vi "main.vi"(11 "Camera":refnum<queue>) -> ()   [LabVIEW 2024, in "RSeries_CAM.lvlib"]
uses:
  RSeries_CAM.lvlib
  ARCH/Message Queue/Message Cluster.ctl
  SRC/SUBVIS/RSeries_CAM.lvclass
  SRC/SUBVIS/RSeries_CAM.lvclass/RSeries_CAM.ctl
  SRC/CTRLS/CAM module Data.ctl
  CTRLS/GLB_VAR.vi
  ARCH/Message Queue/Message Queue.lvlib
panel:
  out "error out 5":errorcluster
  out "error out 4":errorcluster
  out "error out 3":errorcluster
  out "error out":errorcluster
  out "local stop":bool
  out "data out":string
  out "error out 2":errorcluster
  in  "Port 3":u32=3000
  out "RSeries_CAM out":refnum<class "RSeries_CAM.lvclass">
  out "Array":string[](array[string])
  in  "Send Vars":bool
  in  "Cluster":T1
  out "Response":string
  out "Connection status":bool
  in  "Port 2":u32=3001
  in  "Send Command":bool
  in  "Connect":bool
  in  "Command":string
  in  "IP":string="192.168.250.5"
  in  "RSeries_CAM.lvlib:RSeries_CAM.lvclass":refnum<class "RSeries_CAM.lvclass">
  in  "stop":bool
  in  "UNIT TESTING":bool
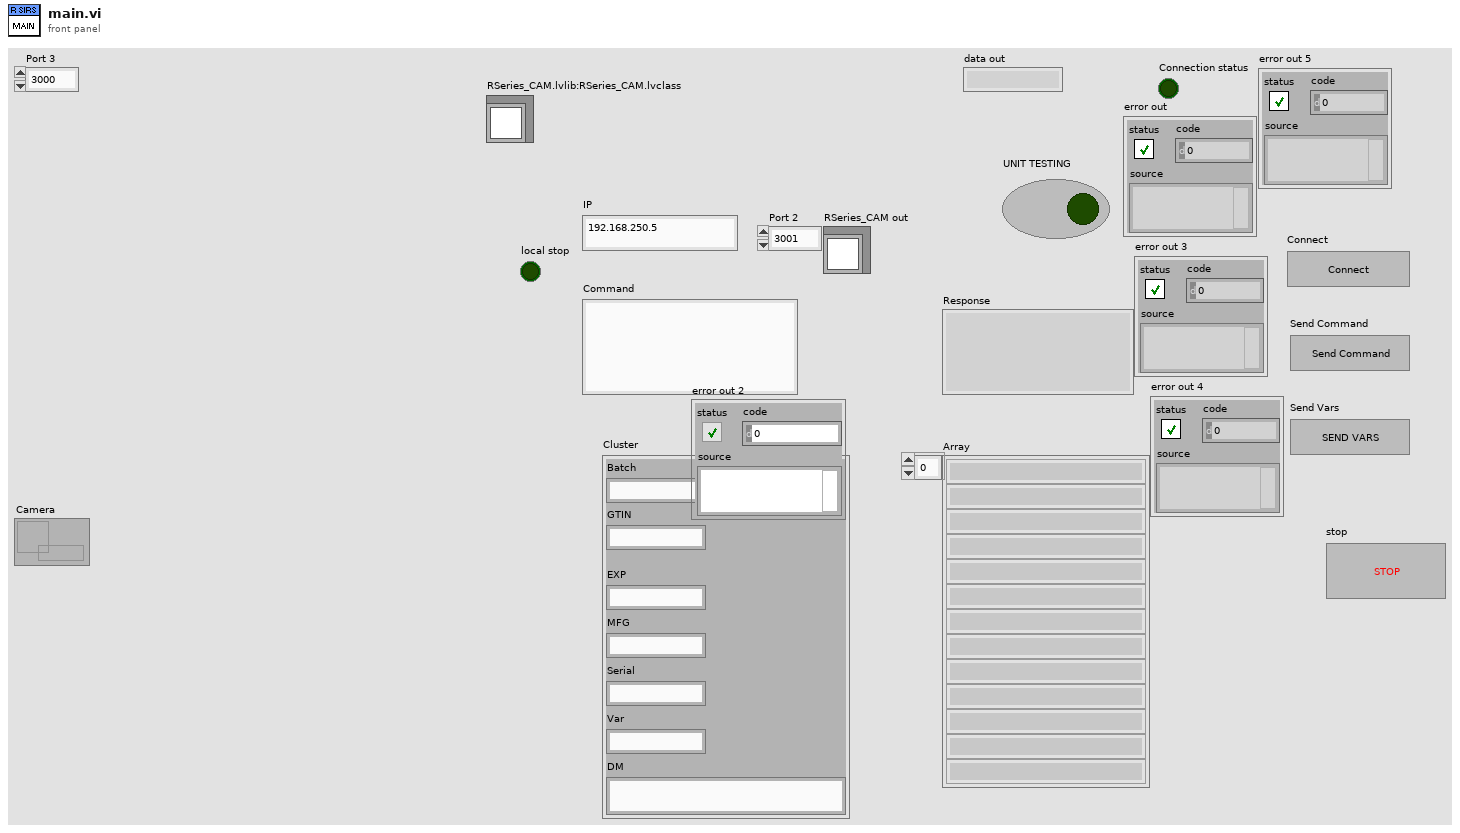
[diagram p1: front panel]
types:
  T1 = cluster{"Batch":string, "GTIN":string, "EXP":string, "MFG":string, "Serial":string, "Var":string, "DM":string}
  T2 = typedef "CAM module Data.ctl" = cluster{"IP":string, "sending Port ":u32, "BatchData":refnum<vi>, "Recieveing Port":u32, "Caller Quue":refnum<queue>}
  T3 = cluster{"Subscriber message":string, "Subscriber queue":refnum<queue>}
  T4 = typedef "Message Queue.lvlib/Message Cluster.ctl" = cluster{"Message":string, "Message Data":variant}
  T5 = enum16{"Standard", "Buffered", "CRLF", "Immediate"}
  T6 = enum16{"Init SRL Buffer", "Insert SRL in Buffer", "Insert SRL Status", "Remove SRL from Buffer", "pop serial"}
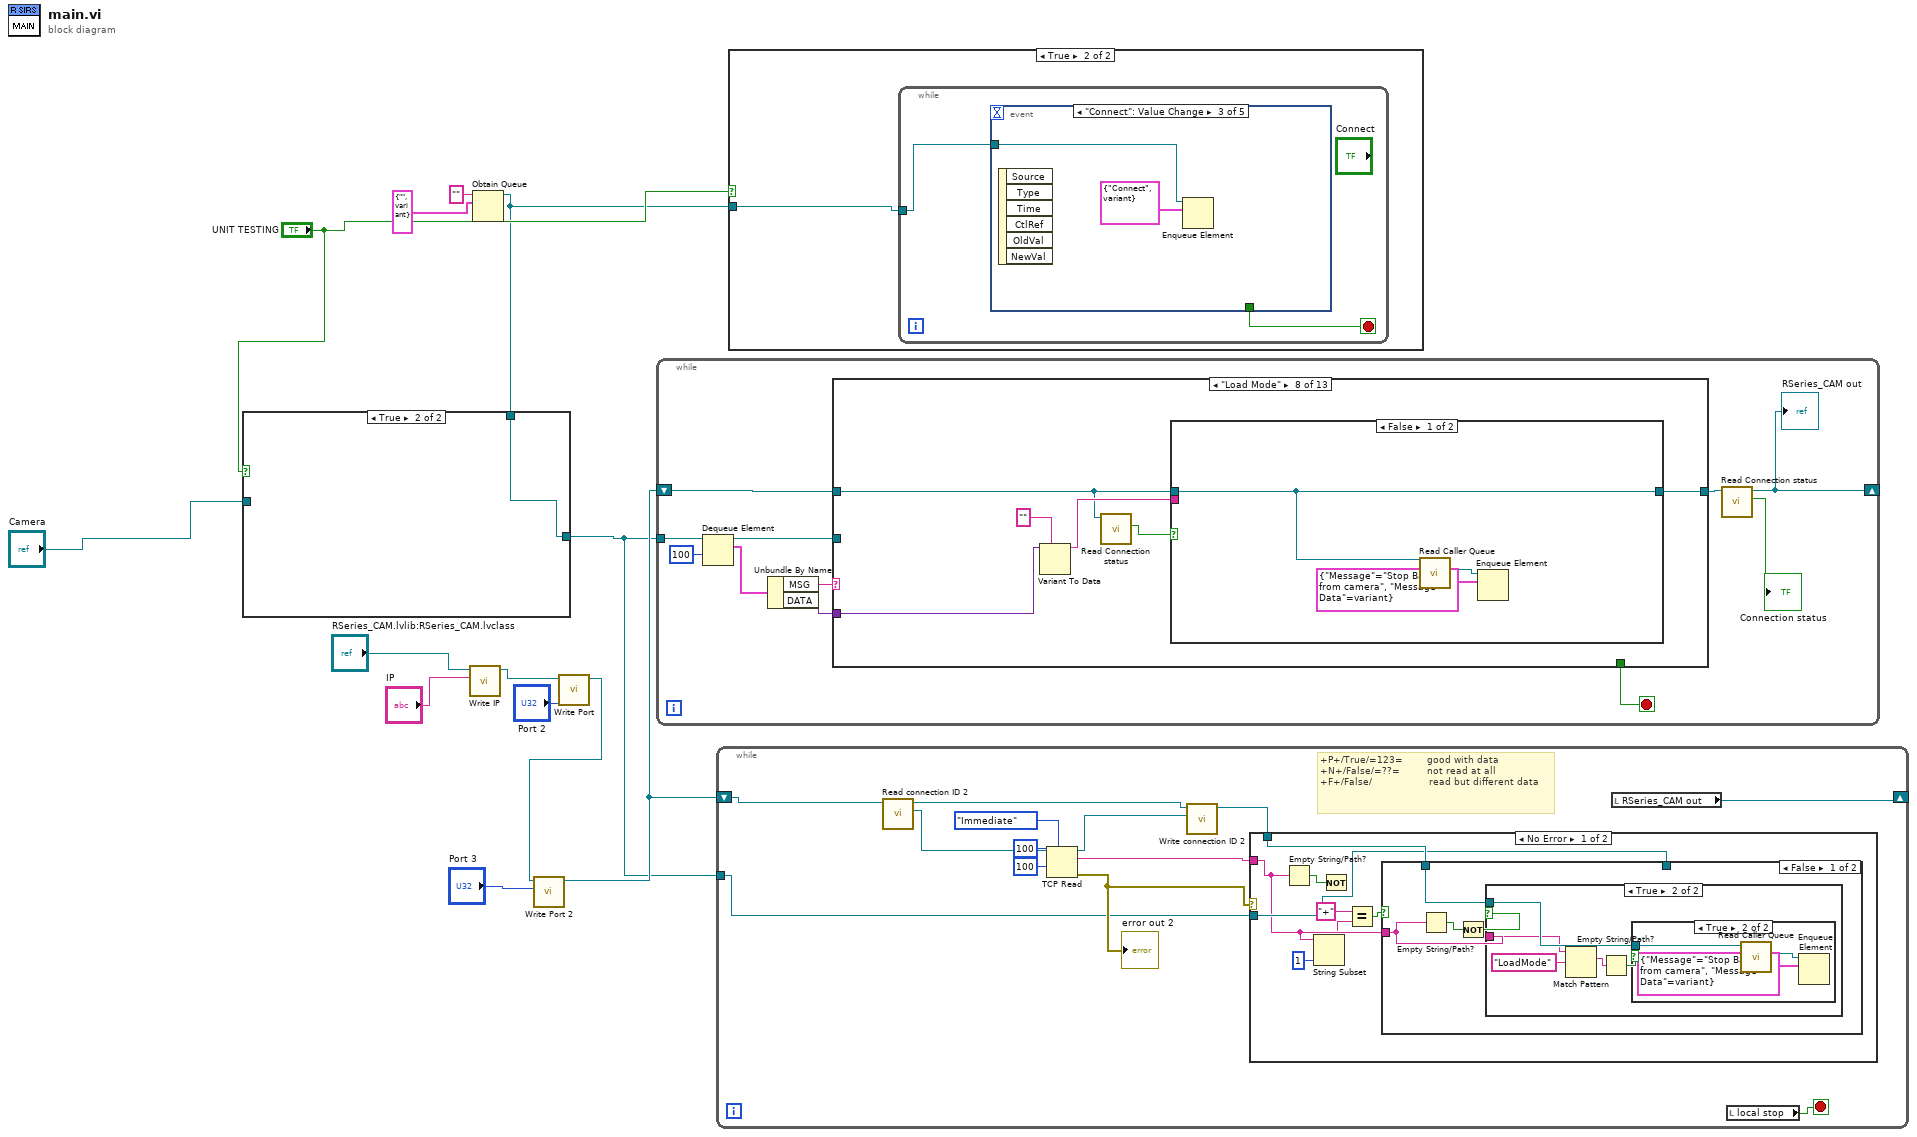
[diagram p0: block diagram]
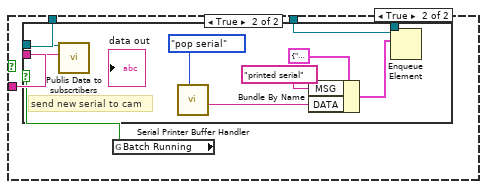
[diagram p4: hidden frame]
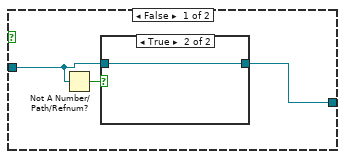
[diagram p7: hidden frame]
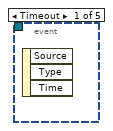
[diagram p10: hidden frame]
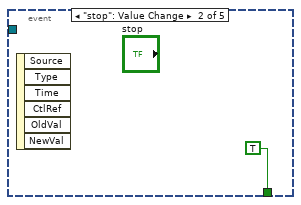
[diagram p11: hidden frame]
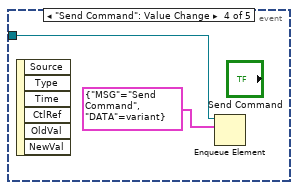
[diagram p12: hidden frame]
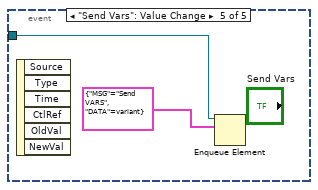
[diagram p13: hidden frame]
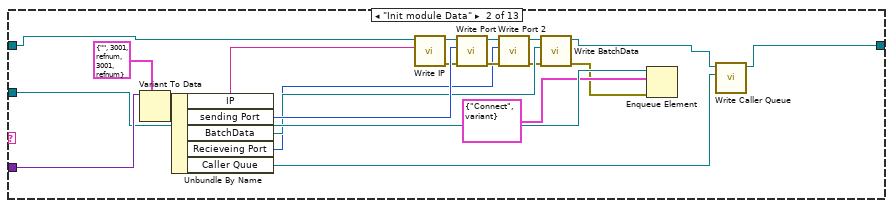
[diagram p15: hidden frame]
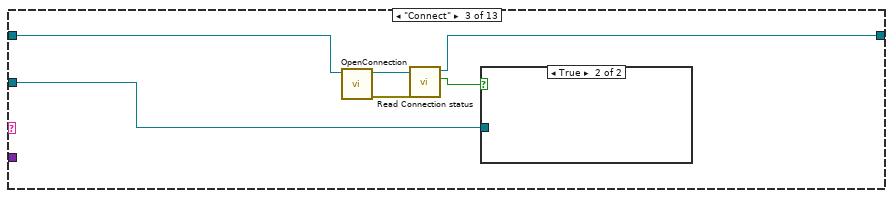
[diagram p16: hidden frame]
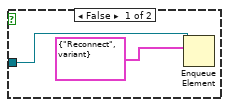
[diagram p17: hidden frame]
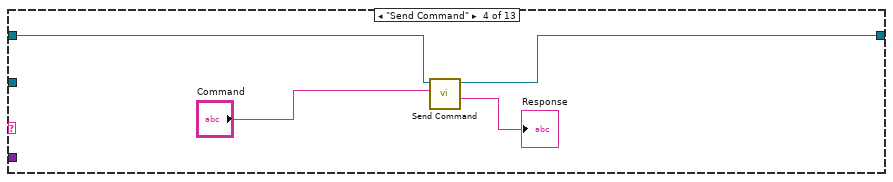
[diagram p18: hidden frame]
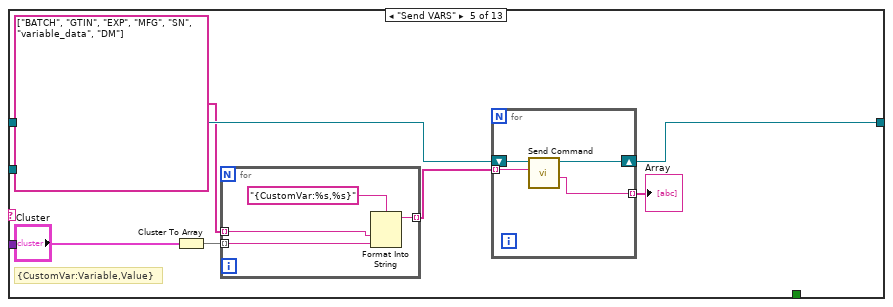
[diagram p19: hidden frame]
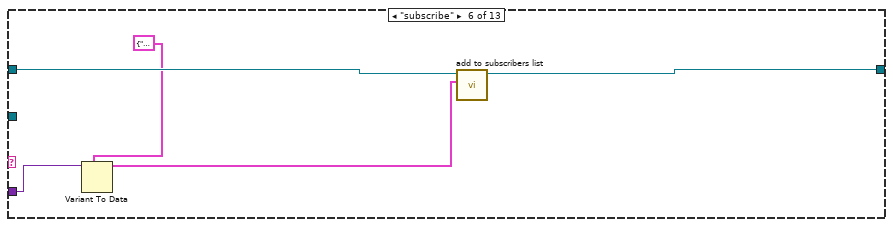
[diagram p20: hidden frame]
diagram:
  n1 = call "Write IP.vi"("IP"="IP", "RSeries_CAM in"="RSeries_CAM.lvlib:RSeries_CAM.lvclass") -> ("RSeries_CAM out"=w7:refnum<class "RSeries_CAM.lvclass">)  [unwired: 8 in, 1 out]
  n2 = Obtain Queue(name (unnamed)="", element data type=cluster{"MSG":string, "DATA":variant} {"MSG"="", "DATA"=variant}) -> (queue out=w9:refnum<queue>)  [unwired: 3 in, 2 out]
  n3 = case shown="True" "UNIT TESTING" {
    tunnel: "Camera" -> [w15 _]
    tunnel: [w14 w19] -> w1
    tunnel: w9 -> [_ w19]
    frame False {
      n4 = Not A Number/Path/Refnum?(number/path/refnum=w15) -> (NaN/Path/Refnum?=w16:bool)
      n5 = case shown="True" w16 {
        tunnel: [w17 w18] -> w14
        tunnel: w15 -> [w17 w18]
        frame False {
        }
        frame True {
        }
      }
    }
    frame True {
    }
  }
  n6 = call "Write Port.vi"("Port"="Port 2", "RSeries_CAM in"=w7) -> ("RSeries_CAM out"=w5:refnum<class "RSeries_CAM.lvclass">)  [unwired: 8 in, 1 out]
  n7 = call "Write Port 2.vi"("Port 2"="Port 3", "RSeries_CAM in"=w5) -> ("RSeries_CAM out"=w4:refnum<class "RSeries_CAM.lvclass">)  [unwired: 8 in, 1 out]
  n8 = while {
    tunnel: w1 -> [w30]
    shift-right: [w20] -> _
    shift-left: w4 -> [w26]
    stop <- w27 stop-if-true
    n9 = Dequeue Element(queue=w30, timeout in ms (-1)=100) -> (queue out=w25:refnum<queue>, element=w29:cluster{"MSG":string, "DATA":variant})  [unwired: 1 in, 2 out]
    n10 = Unbundle By Name(w29) -> ("MSG"=w28:string, "DATA"=w21:variant)
    n11 = case shown="\"Load Mode\"" w28 {
      tunnel: [_ _ _ _ _ _ _ _ _ _ _ _ w151] -> w27
      tunnel: w26 -> [w31 w48 w57 w63 w70 w83 w88 w90 w110 w117 w122 w142 w152]
      tunnel: [w31 w33 w55 w62 w69 w82 w87 w91 w108 w116 w125 w137 w152] -> w24
      tunnel: w25 -> [_ w44 w53 _ _ _ _ _ _ _ w123 w136 _]
      tunnel: w21 -> [_ w51 _ _ _ w81 w86 w92 _ _ w127 _ _]
      frame Default {
      }
      frame "Init module Data" {
        n12 = Variant To Data(type=T2 {"IP"="", "sending Port "=3001, "BatchData"=refnum, "Recieveing Port"=3001, "Caller Quue"=refnum} ("Cluster 2"), Variant=w51) -> (data=w47:T2)  [unwired: 1 in, 1 out]
        n13 = Unbundle By Name(w47) -> ("IP"=w46:string, "sending Port"=w45:u32, "BatchData"=w40:refnum<vi>, "Recieveing Port"=w35:u32, "Caller Quue"=w32:refnum<queue>)
        n14 = call "Write IP.vi"("IP"=w46, "RSeries_CAM in"=w48) -> ("error out"=w42:errorcluster, "RSeries_CAM out"=w49:refnum<class "RSeries_CAM.lvclass">)  [unwired: 8 in]
        n15 = call "Write Port.vi"("error in (no error)"=w42, "Port"=w45, "RSeries_CAM in"=w49) -> ("error out"=w37:errorcluster, "RSeries_CAM out"=w39:refnum<class "RSeries_CAM.lvclass">)  [unwired: 7 in]
        n16 = call "Write Port 2.vi"("error in (no error)"=w37, "Port 2"=w35, "RSeries_CAM in"=w39) -> ("error out"=w36:errorcluster, "RSeries_CAM out"=w38:refnum<class "RSeries_CAM.lvclass">)  [unwired: 7 in]
        n17 = call "Write BatchData.vi"("error in (no error)"=w36, "BatchData"=w40, "RSeries_CAM in"=w38) -> ("error out"=w41:errorcluster, "RSeries_CAM out"=w34:refnum<class "RSeries_CAM.lvclass">)  [unwired: 7 in]
        n18 = Enqueue Element(queue=w44, element=cluster{"MSG":string, "DATA":variant} {"MSG"="Connect", "DATA"=variant}, error in (no error)=w41) -> ()  [unwired: 1 in, 3 out]
        n19 = call "Write Caller Queue.vi"("Caller Queue"=w32, "RSeries_CAM in"=w34) -> ("RSeries_CAM out"=w33:refnum<class "RSeries_CAM.lvclass">)  [unwired: 8 in, 1 out]
      }
      frame "Connect" {
        n20 = call "OpenConnection.vi"("RSeries_CAM in"=w57) -> ("error out"=w52:errorcluster, "RSeries_CAM out"=w56:refnum<class "RSeries_CAM.lvclass">)  [unwired: 9 in]
        n21 = call "Read Connection status.vi"("error in (no error)"=w52, "RSeries_CAM in"=w56) -> ("Connection status"=w54:bool, "RSeries_CAM out"=w55:refnum<class "RSeries_CAM.lvclass">)  [unwired: 7 in, 1 out]
        n22 = case shown="True" w54 {
          tunnel: w53 -> [w58 _]
          frame False {
            n23 = Enqueue Element(queue=w58, element=cluster{"MSG":string, "DATA":variant} {"MSG"="Reconnect", "DATA"=variant}) -> ()  [unwired: 2 in, 3 out]
          }
          frame True {
          }
        }
      }
      frame "Send Command" {
        n24 = call "Send Command.vi"("Command"="Command", "RSeries_CAM in"=w63) -> ("Response"=→"Response":string, "RSeries_CAM out"=w62:refnum<class "RSeries_CAM.lvclass">)  [unwired: 6 in, 2 out]
      }
      frame "Send VARS" {
        # "{CustomVar:Variable,Value}"
        n25 = Cluster To Array(cluster="Cluster") -> (array=w68:string[])
        n26 = for {
          tunnel: string[] ["BATCH", "GTIN", "EXP", "MFG", "SN", "variable_data", "DM"] -> [w78] mode=indexing
          tunnel: w68 -> [w77] mode=indexing
          tunnel: [w75] -> w65 mode=indexing
          n27 = Format Into String(format string="{CustomVar:%s,%s}", w78, w77) -> (resulting string=w75:string)  [unwired: 2 in, 1 out]
        }
        n28 = for {
          shift-right: [w73] -> w69
          shift-left: w70 -> [w74]
          tunnel: w65 -> [w72] mode=indexing
          tunnel: [w71] -> w64 mode=indexing
          n29 = call "Send Command.vi"("Command"=w72, "RSeries_CAM in"=w74) -> ("Response"=w71:string, "RSeries_CAM out"=w73:refnum<class "RSeries_CAM.lvclass">)  [unwired: 6 in, 2 out]
        }
        "Array" <- w64
      }
      frame "subscribe" {
        n30 = Variant To Data(type=T3 {"Subscriber message"="", "Subscriber queue"=refnum} ("Subscriber Data"), Variant=w81) -> (data=w79:T3)  [unwired: 1 in, 1 out]
        n31 = call "add to subscribers list.vi"("Subscriber Data"=w79, "RSeries_CAM in"=w83) -> ("RSeries_CAM out"=w82:refnum<class "RSeries_CAM.lvclass">)  [unwired: 8 in, 1 out]
      }
      frame "unsubscribe" {
        n32 = Variant To Data(type=T3 {"Subscriber message"="", "Subscriber queue"=refnum} ("Subscriber Data"), Variant=w86) -> (data=w84:T3)  [unwired: 1 in, 1 out]
        n33 = call "remove from subscribers list.vi"("Subscriber Data"=w84, "RSeries_CAM in"=w88) -> ("RSeries_CAM out"=w87:refnum<class "RSeries_CAM.lvclass">)  [unwired: 8 in, 1 out]
      }
      frame "Load Mode" {
        n34 = Variant To Data(type="", Variant=w92) -> (data=w94:string)  [unwired: 1 in, 1 out]
        n35 = call "Read Connection status.vi"("RSeries_CAM in"=w90) -> ("Connection status"=w89:bool)  [unwired: 8 in, 2 out]
        n36 = case shown="False" w89 {
          tunnel: w94 -> [_ w102]
          tunnel: w90 -> [w97 w101]
          tunnel: [w97 w99] -> w91
          frame False {
            n37 = call "Read Caller Queue.vi"("RSeries_CAM in"=w97) -> ("Caller Queue"=w96:refnum<queue>)  [unwired: 8 in, 2 out]
            n38 = Enqueue Element(queue=w96, element=T4 {"Message"="Stop Batch from camera", "Message Data"=variant}) -> ()  [unwired: 2 in, 3 out]
          }
          frame True {
            # "LoadMode:ModeName}"
            n39 = call "LoadMode.vi"("mode name"=w102, "RSeries_CAM in"=w101) -> ("error out"=→"error out 4":errorcluster, "Success?"=w100:bool, "RSeries_CAM out"=w99:refnum<class "RSeries_CAM.lvclass">)  [unwired: 7 in]
            n40 = case shown="False" w100 {
              tunnel: w99 -> [w103 _]
              frame False {
                n41 = disable-structure shown="Disabled" {
                  disable-tunnel: w103 -> [w104 _]
                  frame Disabled {
                    n42 = call "Read Caller Queue.vi"("RSeries_CAM in"=w104) -> ("Caller Queue"=w106:refnum<queue>)  [unwired: 8 in, 2 out]
                    n43 = Enqueue Element(queue=w106, element=T4 {"Message"="Stop Batch from camera", "Message Data"=variant}) -> ()  [unwired: 2 in, 3 out]
                  }
                  frame Enabled {
                  }
                }
              }
              frame True {
              }
            }
          }
        }
      }
      frame "start mode" {
        n44 = call "Start Mode.vi"("RSeries_CAM in"=w110) -> ("error out"=→"error out 3":errorcluster, "Success?"=w109:bool, "RSeries_CAM out"=w108:refnum<class "RSeries_CAM.lvclass">)  [unwired: 8 in]
        n45 = case shown="False" w109 {
          tunnel: w108 -> [w111 _]
          frame False {
            n46 = disable-structure shown="Disabled" {
              disable-tunnel: w111 -> [w114 _]
              frame Disabled {
                n47 = call "Read Caller Queue.vi"("RSeries_CAM in"=w114) -> ("Caller Queue"=w113:refnum<queue>)  [unwired: 8 in, 2 out]
                n48 = Enqueue Element(queue=w113, element=T4 {"Message"="Stop Batch", "Message Data"=variant}) -> ()  [unwired: 2 in, 3 out]
              }
              frame Enabled {
              }
            }
          }
          frame True {
          }
        }
      }
      frame "stop mode" {
        n49 = call "StopMode.vi"("RSeries_CAM in"=w117) -> ("error out"=→"error out":errorcluster, "RSeries_CAM out"=w116:refnum<class "RSeries_CAM.lvclass">)  [unwired: 8 in, 1 out]
      }
      frame "printed serial" {
        n50 = Variant To Data(type="", Variant=w127) -> (data=w119:string)  [unwired: 1 in, 1 out]
        n51 = call "encode DM.vi"("serial"=w119, "RSeries_CAM in"=w122) -> ("DM"=w120:string, "RSeries_CAM out"=w121:refnum<class "RSeries_CAM.lvclass">)  [unwired: 7 in, 1 out]
        n52 = call "Insert Custom Var.vi"("Value"=w120, "Var Name"="dm", "RSeries_CAM in"=w121) -> ("error out"=→"error out 5":errorcluster, "Success?"=w124:bool, "RSeries_CAM out"=w125:refnum<class "RSeries_CAM.lvclass">)  [unwired: 6 in]
        n53 = case shown="False" w124 {
          tunnel: w123 -> [w130 _]
          tunnel: w119 -> [w129 _]
          frame False {
            n54 = disable-structure shown="Disabled" {
              disable-tunnel: w130 -> [w135 _]
              disable-tunnel: w129 -> [w134 _]
              frame Disabled {
                n55 = Bundle By Name(cluster=cluster{"MSG":string, "DATA":variant} {"MSG"="", "DATA"=variant} ("element"), "MSG"="printed serial", "DATA"=w134) -> (w131:cluster{"MSG":string, "DATA":variant})
                n56 = Enqueue Element(queue=w135, element=w131) -> ()  [unwired: 2 in, 3 out]
              }
              frame Enabled {
              }
            }
          }
          frame True {
          }
        }
      }
      frame "Reconnect" {
        n57 = flat-sequence {
          tunnel: w142 -> [w146]
          tunnel: [w145] -> w141
          tunnel: w141 -> [w147]
          tunnel: [w147] -> w140
          tunnel: w140 -> [w150]
          tunnel: [w149] -> w138
          frame #0 {
            n58 = call "Disconnect.vi"("RSeries_CAM in"=w146) -> ("RSeries_CAM out"=w145:refnum<class "RSeries_CAM.lvclass">)  [unwired: 9 in, 1 out]
          }
          frame #1 {
            n59 = Wait (ms)(milliseconds to wait=u32 500) -> ()  [unwired: 1 out]
          }
          frame #2 {
            n60 = call "OpenConnection.vi"("RSeries_CAM in"=w150) -> ("RSeries_CAM out"=w149:refnum<class "RSeries_CAM.lvclass">)  [unwired: 9 in, 1 out]
          }
        }
        n61 = call "Read Connection status.vi"("RSeries_CAM in"=w138) -> ("Connection status"=w139:bool, "RSeries_CAM out"=w137:refnum<class "RSeries_CAM.lvclass">)  [unwired: 8 in, 1 out]
        n62 = case shown="False" w139 {
          tunnel: w136 -> [w143 _]
          frame False {
            n63 = Enqueue Element(queue=w143, element=cluster{"MSG":string, "DATA":variant} {"MSG"="Reconnect", "DATA"=variant}) -> ()  [unwired: 2 in, 3 out]
          }
          frame True {
          }
        }
      }
      frame "Exit" {
        w151 = TRUE
        "local stop" <- w151
      }
    }
    n64 = call "Read Connection status.vi"("RSeries_CAM in"=w24) -> ("Connection status"=→"Connection status":bool, "RSeries_CAM out"=w20:refnum<class "RSeries_CAM.lvclass">)  [unwired: 8 in, 1 out]
    "RSeries_CAM out" <- w20
  }
  n65 = while {
    shift-right: [w160] -> _
    shift-left: w4 -> [w159]
    tunnel: w1 -> [w153]
    stop <- w155 stop-if-true
    # "+P+/True/=123=        good with data\n+N+/False/=??=         not read at all\n+F+/False/                   read but different data"
    n66 = call "Read connection ID 2.vi"("RSeries_CAM in"=w159) -> ("connection ID 2"=w158:refnum<k5>, "RSeries_CAM out"=w156:refnum<class "RSeries_CAM.lvclass">)  [unwired: 8 in, 1 out]
    n67 = TCP Read(connection ID=w158, bytes to read=100, 7:T5."Immediate" ("mode (standard)"), 9:100 ("timeout ms (25000)")) -> (connection ID out=w157:refnum<k5>, data out=w165:string, error out=w164:errorcluster)  [unwired: 1 in]
    "error out 2" <- w164
    n68 = call "Write connection ID 2.vi"("connection ID 2"=w157, "RSeries_CAM in"=w156) -> ("RSeries_CAM out"=w154:refnum<class "RSeries_CAM.lvclass">)  [unwired: 8 in, 1 out]
    n69 = case shown="No Error" w164 {
      tunnel: w165 -> [w169 _]
      tunnel: w154 -> [w172 _]
      tunnel: w153 -> [w171 _]
      frame No Error {
        n70 = Empty String/Path?(string/path=w169) -> (empty?=w173:bool)
        n71 = String Subset(string=w169, length (rest)=1 ("length (rest)")) -> (substring=w168:string)  [unwired: 1 in]
        n72 = Not(x=w173) -> ()  [unwired: 1 out]
        n73 = Equal?(x="+", y=w168) -> (x = y?=w166:bool)
        n74 = case shown="False" w166 {
          tunnel: w169 -> [w174 w189]
          tunnel: w172 -> [w175 w188]
          tunnel: w171 -> [_ w187]
          frame False {
            n75 = Empty String/Path?(string/path=w174) -> (empty?=w177:bool)
            n76 = Not(x=w177) -> (.not. x?=w176:bool)
            n77 = case shown="True" w176 {
              tunnel: w175 -> [_ w182]
              tunnel: w174 -> [_ w181]
              frame False {
              }
              frame True {
                n78 = Match Pattern(string=w181, regular expression="LoadMode") -> (match substring=w179:string)  [unwired: 1 in, 3 out]
                n79 = Empty String/Path?(string/path=w179) -> (empty?=w178:bool)
                n80 = case shown="True" w178 {
                  tunnel: w182 -> [_ w183]
                  frame False {
                  }
                  frame True {
                    n81 = call "Read Caller Queue.vi"("RSeries_CAM in"=w183) -> ("Caller Queue"=w185:refnum<queue>)  [unwired: 8 in, 2 out]
                    n82 = Enqueue Element(queue=w185, element=T4 {"Message"="Stop Batch from camera", "Message Data"=variant}) -> ()  [unwired: 2 in, 3 out]
                  }
                }
              }
            }
          }
          frame True {
            n83 = global read "GLB_VAR.vi" "Batch Running"() -> (w186:bool)
            n84 = case shown="True" w186 {
              tunnel: w189 -> [_ w197]
              tunnel: w188 -> [_ w196]
              tunnel: w187 -> [_ w191]
              frame False {
              }
              frame True {
                # "send new serial to cam"
                n85 = call "Publis Data to subscrtibers.vi"("Message Data"=w197, "RSeries_CAM in"=w196) -> ()  [unwired: 8 in, 2 out]
                n86 = call "Serial Printer Buffer Handler.vi"("Serials buffer operations"=T6."pop serial") -> ("poped serial"=w190:string)  [unwired: 9 in, 1 out]
                n87 = Bundle By Name(cluster=cluster{"MSG":string, "DATA":variant} {"MSG"="", "DATA"=variant} ("element"), "MSG"="printed serial", "DATA"=w190) -> (w192:cluster{"MSG":string, "DATA":variant})
                n88 = Enqueue Element(queue=w191, element=w192) -> ()  [unwired: 2 in, 3 out]
              }
            }
          }
        }
      }
      frame Error {
      }
    }
    n89 = local read "RSeries_CAM out"() -> (w160:refnum<class "RSeries_CAM.lvclass">)
    n90 = local read "local stop"() -> (w155:bool)
  }
  n91 = case shown="True" "UNIT TESTING" {
    tunnel: w9 -> [_ w198]
    frame False {
    }
    frame True {
      n92 = while {
        tunnel: w198 -> [w199]
        stop <- w200 stop-if-true
        n93 = event shown="[2] \"Connect\": Value Change" {
          selector: _ -> [_ _ _ _ _]
          dyn-events: _ -> [_ _ _ _ _]
          timeout: _ -> [_ _ _ _ _]
          tunnel: [_ TRUE _ _ _] -> w200
          tunnel: w199 -> [_ _ w203 w204 w206]
          event Timeout {
            n94 = event-data() -> ()  [unwired: 1 in, 3 out]
          }
          event "stop": Value Change {
            n95 = event-data() -> ()  [unwired: 1 in, 6 out]
          }
          event "Connect": Value Change {
            n96 = event-data() -> ()  [unwired: 1 in, 6 out]
            n97 = Enqueue Element(queue=w203, element=cluster{"MSG":string, "DATA":variant} {"MSG"="Connect", "DATA"=variant}) -> ()  [unwired: 2 in, 3 out]
          }
          event "Send Command": Value Change {
            n98 = event-data() -> ()  [unwired: 1 in, 6 out]
            n99 = Enqueue Element(queue=w204, element=cluster{"MSG":string, "DATA":variant} {"MSG"="Send Command", "DATA"=variant}) -> ()  [unwired: 2 in, 3 out]
          }
          event "Send Vars": Value Change {
            n100 = event-data() -> ()  [unwired: 1 in, 6 out]
            n101 = Enqueue Element(queue=w206, element=cluster{"MSG":string, "DATA":variant} {"MSG"="Send VARS", "DATA"=variant}) -> ()  [unwired: 2 in, 3 out]
          }
        }
      }
    }
  }
